vi "Export ConPanes.vi"() -> ()   [LabVIEW 2021]
panel:
  out "Name":string
  out "Error":errorcluster
  in  "Images Dir":path=path "C:/Projects/LabVIEW/RyLibs/ry.lib/ryTimer/Help/Images"
  in  "Library Path":path=path "C:/Projects/LabVIEW/RyLibs/ry.lib/ryTimer/Lib/ryTimer.lvclass"
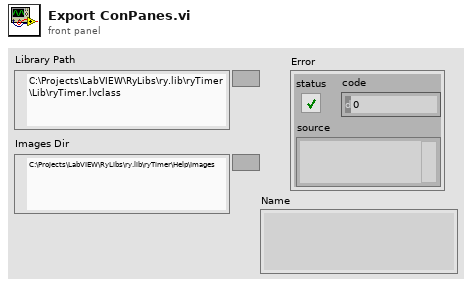
[diagram p1: front panel]
types:
  T1 = enum32{"invalid VI type", "Standard VI", "Control VI", "Global VI", "Polymorphic VI", "Configuration VI", "SubSystem", "Facade VI", "Method VI", "Statechart Diagram VI"}
  T2 = typedef "imagedata.ctl" = cluster{"image type":i32, "image depth":i32, "image":u8[], "mask":u8[], "colors":u32[], "Rectangle":cluster{"left":i16, "top":i16, "right":i16, "bottom":i16}}
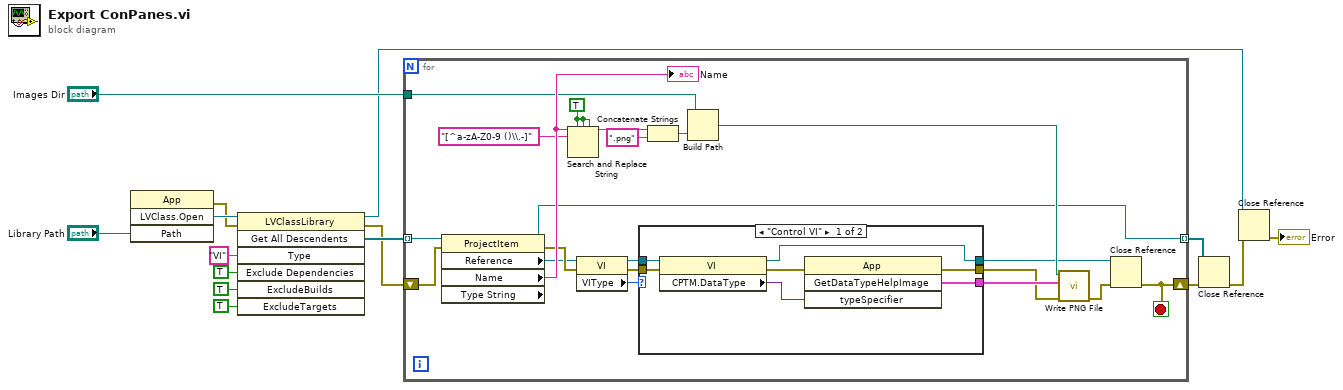
[diagram p0: block diagram]
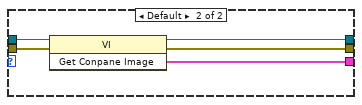
[diagram p2: hidden frame]
diagram:
  n1 = invoke class="App" method="LVClass.Open"("Path"="Library Path") -> (error out=w13:errorcluster, "LVClass.Open"=w14:refnum<vi>)  [unwired: 3 in, 2 out]
  n2 = invoke class="LVClassLibrary" method="Get All Descendents"(reference=w14, error in=w13, "Type"="VI", "Exclude Dependencies"=TRUE ("ExcludeDependencies"), "ExcludeBuilds"=TRUE, "ExcludeTargets"=TRUE) -> (reference out=w3:refnum<vi>, error out=w7:errorcluster, "All Descendents"=w8:refnum<vi>[])  [unwired: 1 in, 4 out]
  n3 = for {
    tunnel: w8 -> [w36] mode=indexing
    tunnel: "Images Dir" -> [w29]
    tunnel: [w17] -> w4 mode=indexing
    shift-right: [w23] -> w5
    shift-left: w7 -> [w35]
    stop <- w23 stop-if-true
    w32 = TRUE ("replace all? (F)")
    n4 = property class="ProjectItem" props=["Reference", "Name", "Type String"](reference=w36, error in=w35) -> (reference out=w17:refnum<vi>, error out=w21:errorcluster, "Reference"=w19:refnum<vi>, "Name"=w33:string)  [unwired: 1 out]
    "Name" <- w33
    n5 = Search and Replace String(replace all?=w32, case sensitive?=w32, multiline?=w32, input string=w33, search string="[^a-zA-Z0-9 ()\\.-]") -> (result string=w30:string)  [unwired: 3 in, 3 out]
    n6 = property class="VI"(reference=w19, error in=w21) -> (reference out=w18:refnum<vi>, error out=w20:errorcluster, "VIType"=w16:T1)
    n7 = case shown="\"Control VI\"" w16 {
      tunnel: [w39 w48] -> w34
      tunnel: [w38 w47] -> w25
      tunnel: [w37 w46] -> w22
      tunnel: w20 -> [w43 w45]
      tunnel: w18 -> [w42 w44]
      frame "Control VI" {
        n8 = property class="VI"(reference=w42, error in=w43) -> (reference out=w37:refnum<vi>, error out=w41:errorcluster, "CPTM.DataType"=w40:variant)
        n9 = invoke class="App" method="GetDataTypeHelpImage"(error in=w41, "typeSpecifier"=w40) -> (error out=w38:errorcluster, "GetDataTypeHelpImage"=w39:T2)  [unwired: 2 in, 2 out]
      }
      frame Default {
        n10 = invoke class="VI" method="Get Conpane Image"(reference=w44, error in=w45) -> (reference out=w46:refnum<vi>, error out=w47:errorcluster, "Get Conpane Image"=w48:T2)  [unwired: 1 in]
      }
    }
    n11 = Concatenate Strings(w30, ".png" ("string")) -> (w28:string)
    n12 = Build Path(base path=w29, name or relative path=w28) -> (appended path=w26:path)
    n13 = call <vilib>:"Write PNG File.vi"("error in (no error)"=w25, "image data"=w34, "path to PNG file"=w26) -> ("error out"=w24:errorcluster)  [unwired: 7 in, 1 out]
    n14 = Close Reference(reference=w22, error in (no error)=w24) -> (error out=w23:errorcluster)
  }
  n15 = Close Reference(reference=w4, error in (no error)=w5) -> (error out=w2:errorcluster)
  n16 = Close Reference(reference=w3, error in (no error)=w2) -> (error out=→"Error":errorcluster)
